vi "User_Login.vi"() -> ()   [LabVIEW 2020]
uses:
  <vilib>/Utility/cursorutil.llb/Set Cursor (Icon Pict).vi
panel:
  in  "Register":bool
  in  "Login":bool
  in  "User_Password":string caption="密    码"
  in  "User_Name":string caption="用户名"
  # "登录系统"
  # "@DTWAVES"
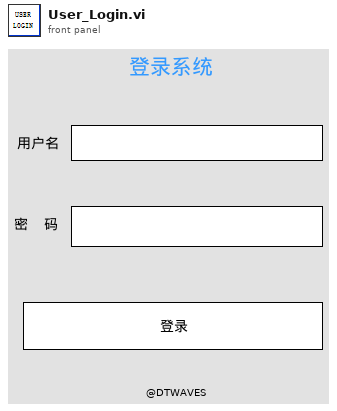
[diagram p1: front panel]
types:
  T1 = enum32{"Invalid", "Standard", "Closed", "Hidden", "Minimized", "Maximized"}
  T2 = enum32{"invalid app kind", "Development System", "Run Time System", "Student Edition", "Embedded LabVIEW", "Evaluation", "Custom"}
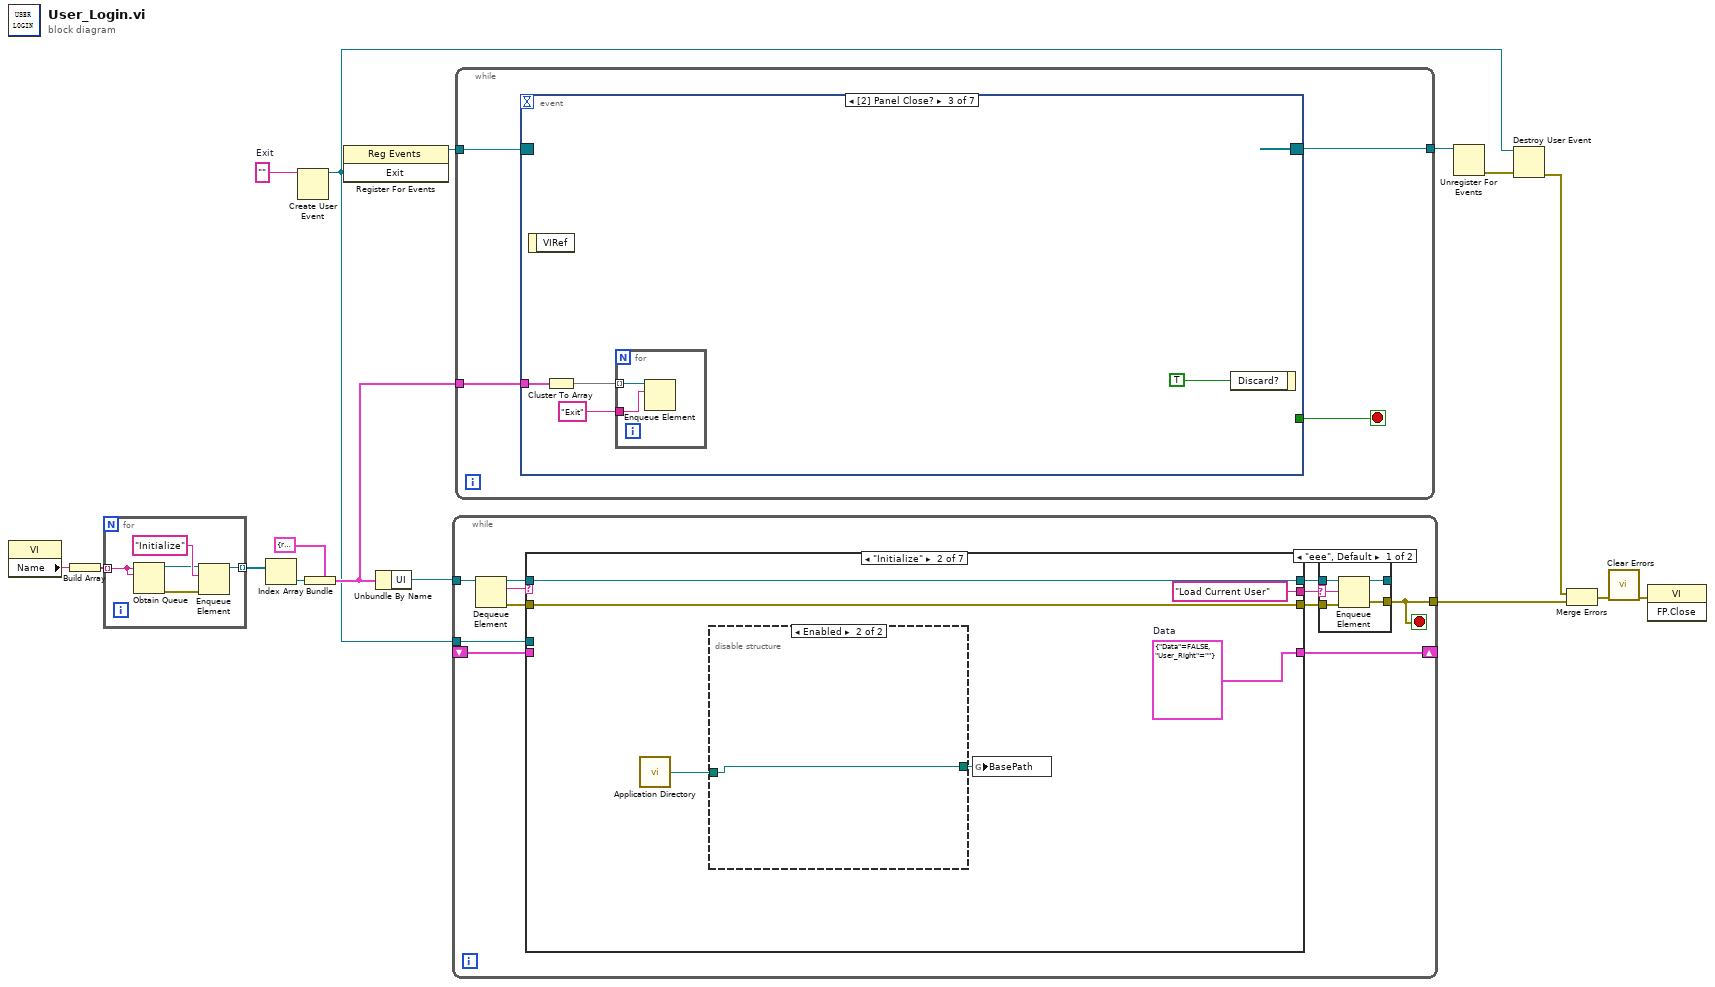
[diagram p0: block diagram]
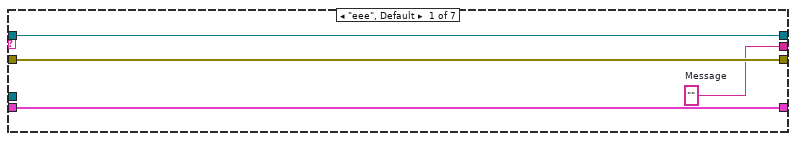
[diagram p3: hidden frame]
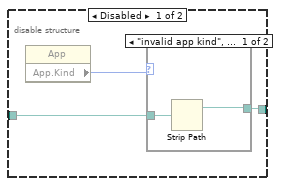
[diagram p4: hidden frame]
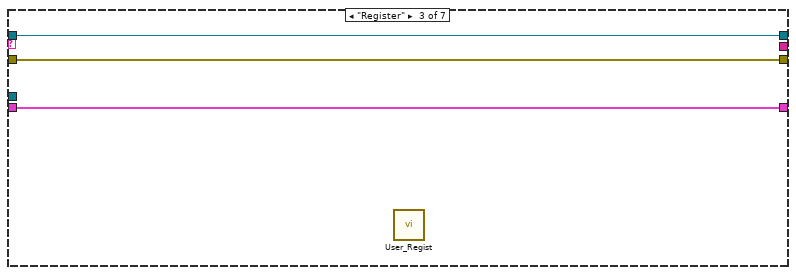
[diagram p6: hidden frame]
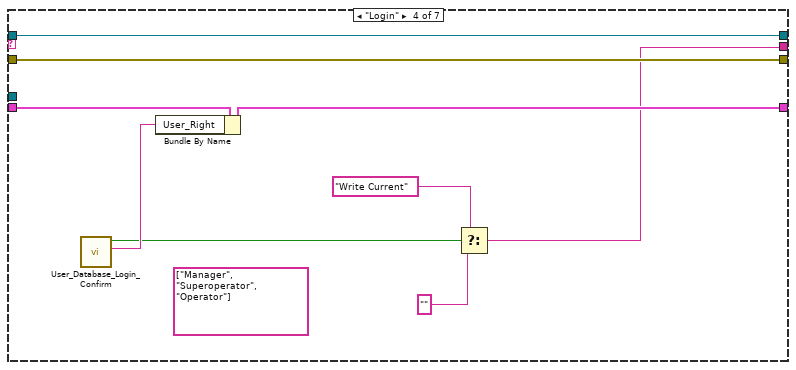
[diagram p7: hidden frame]
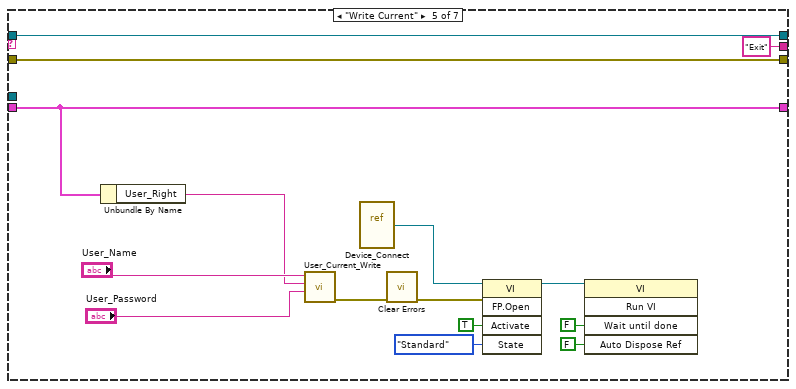
[diagram p8: hidden frame]
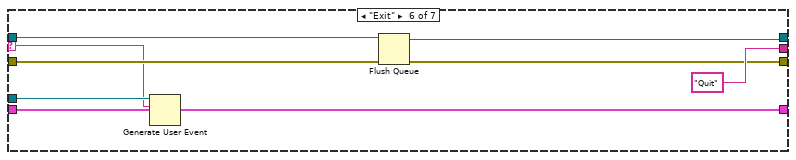
[diagram p9: hidden frame]
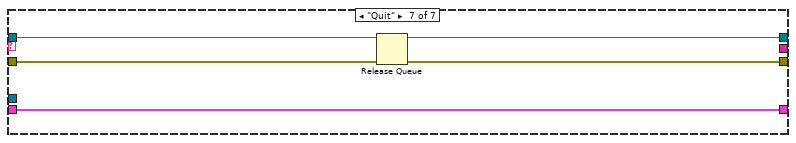
[diagram p10: hidden frame]
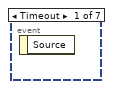
[diagram p11: hidden frame]
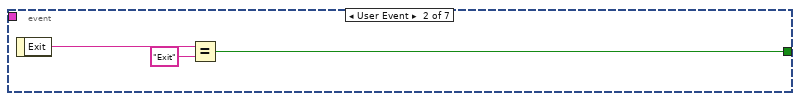
[diagram p12: hidden frame]
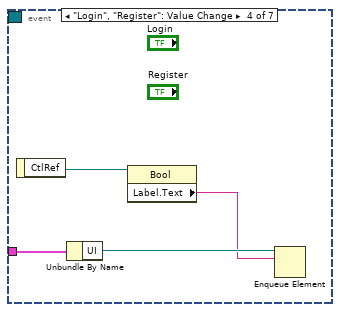
[diagram p13: hidden frame]
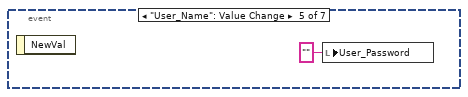
[diagram p14: hidden frame]
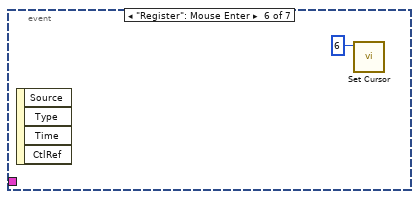
[diagram p15: hidden frame]
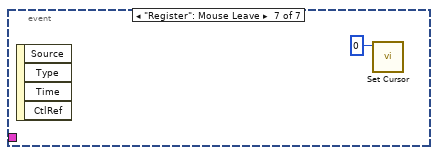
[diagram p16: hidden frame]
diagram:
  w2 = ""  # Exit
  n1 = property class="VI"() -> ("Name"=w12:string)  [unwired: 2 in, 2 out]
  n2 = Build Array(w12) -> (w13:string[])
  n3 = for {
    tunnel: w13 -> [w17] mode=indexing
    tunnel: [w18] -> w7 mode=indexing
    n4 = Obtain Queue(name (unnamed)=w17, element data type=w17) -> (queue out=w20:refnum<queue>, error out=w19:errorcluster)  [unwired: 3 in, 1 out]
    n5 = Enqueue Element(queue=w20, element="Initialize" ("元素"), error in (no error)=w19) -> (queue out=w18:refnum<queue>)  [unwired: 1 in, 2 out]
  }
  n6 = Index Array(array=w7) -> (element=w10:refnum<queue>)  [unwired: 1 in]
  n7 = Create User Event(user event datatype=w2) -> (user event=w6:refnum<user-event>)  [unwired: 1 in, 1 out]
  n8 = Bundle(cluster=cluster{"UI":refnum<queue>} {"UI"=refnum}, "UI"=w10) -> (w11:cluster{"UI":refnum<queue>})
  n9 = register-events(w6) -> (reference out=w3:refnum<event-registration>)  [unwired: 2 in, 1 out]
  n10 = Unbundle By Name(w11) -> ("UI"=w8:refnum<queue>)
  n11 = while {
    tunnel: w8 -> [w32]
    tunnel: [w22] -> w15
    shift-right: [w26] -> _
    shift-left: _ -> [w25]
    tunnel: w6 -> [w24]
    stop <- w22 stop-if-true
    n12 = Dequeue Element(queue=w32) -> (queue out=w31:refnum<queue>, element=w23:string, error out=w28:errorcluster)  [unwired: 2 in, 1 out]
    n13 = case shown="\"Initialize\"" w23 {
      selector: w23 -> [_ _ _ _ _ w84 _]
      tunnel: w31 -> [w43 w49 w59 w68 w83 w89 w95]
      tunnel: [w43 w49 w59 w68 w83 w88 w95] -> w30
      tunnel: [w42 w48 w58 w67 w82 w87 w92] -> w29
      tunnel: w28 -> [w42 w48 w58 w67 w82 w86 w94]
      tunnel: [w41 "Load Current User" ("Message") _ w60 "Exit" ("Message") "Quit" ("Message") _] -> w27
      tunnel: [w40 w47 w57 w65 w80 w91 w93] -> w26
      tunnel: w25 -> [w40 _ w57 w66 w80 w91 w93]
      tunnel: w24 -> [_ _ _ _ _ w85 _]
      frame "eee", Default {
        w41 = ""  # Message
      }
      frame "Initialize" {
        w47 = cluster{"Data":bool, "User_Right":string} {"Data"=FALSE, "User_Right"=""}  # Data
        n14 = call <vilib>:"Application Directory.vi"() -> ("Application Directory"=w45:path)
        n15 = disable-structure shown="Enabled" {
          disable-tunnel: w45 -> [w51 w56]
          disable-tunnel: [w50 w56] -> w44
          frame Disabled {
            n16 = property class="App"() -> ("App.Kind"=w52:T2)  [unwired: 2 in, 2 out]
            n17 = case shown="\"invalid app kind\", Default" w52 {
              tunnel: [w53 w55] -> w50
              tunnel: w51 -> [w54 w55]
              frame "invalid app kind", Default {
                n18 = Strip Path(path=w54) -> (stripped path=w53:path)  [unwired: 1 out]
              }
              frame "Development System" {
              }
            }
          }
          frame Enabled {
          }
        }
        n19 = global write "Global.vi" "BasePath"(w44) -> ()
      }
      frame "Register" {
        n20 = call "User_Regist.vi"() -> ()  [unwired: 12 in]
      }
      frame "Login" {
        (unwired) string[] ["Manager", "Superoperator", "Operator"] ("字符串数组")
        n21 = call "User_Database_Login_Confirm.vi"() -> ("User_Right"=w64:string, "OK"=w63:bool)  [unwired: 9 in, 1 out]
        n22 = Bundle By Name(cluster=w66, "User_Right"=w64) -> (w65:cluster{"Data":bool, "User_Right":string})
        n23 = Select(t="Write Current", s=w63, f="") -> (s? t:f=w60:string)
      }
      frame "Write Current" {
        n24 = Unbundle By Name(w80) -> ("User_Right"=w76:string)
        n25 = call "User_Current_Write.vi"("Password"="User_Password", "User_Right"=w76, "Name"="User_Name") -> ("error out"=w79:errorcluster)  [unwired: 8 in]
        n26 = vi-ref "Device_Connect.vi"() -> (w74:refnum<vi>)
        n27 = call <vilib>:"Clear Errors.vi"("error in (no error)"=w79) -> ("error out"=w69:errorcluster)  [unwired: 5 in, 1 out]
        n28 = invoke class="VI" method="FP.Open"(reference=w74, error in=w69, "Activate"=TRUE ("激活？"), "State"=T1."Standard" ("状态")) -> (reference out=w75:refnum<vi>)  [unwired: 1 in, 4 out]
        n29 = invoke class="VI" method="Run VI"(reference=w75, "Wait until done"=FALSE ("结束前等待"), "Auto Dispose Ref"=FALSE ("自动销毁引用")) -> ()  [unwired: 2 in, 5 out]
      }
      frame "Exit" {
        n30 = Generate User Event(user event=w85, event data cluster=w84) -> ()  [unwired: 2 in, 2 out]
        n31 = Flush Queue(queue=w89, error in (no error)=w86) -> (queue out=w88:refnum<queue>, error out=w87:errorcluster)  [unwired: 1 out]
      }
      frame "Quit" {
        n32 = Release Queue(queue=w95, error in (no error)=w94) -> (error out=w92:errorcluster)  [unwired: 1 in, 2 out]
      }
    }
    n33 = case shown="\"eee\", Default" w27 {
      selector: w27 -> [w33 _]
      tunnel: w30 -> [w37 w39]
      tunnel: w29 -> [w36 w38]
      tunnel: [w35 w38] -> w22
      tunnel: [w34 w39] -> _
      frame "eee", Default {
        n34 = Enqueue Element(queue=w37, element=w33, error in (no error)=w36) -> (queue out=w34:refnum<queue>, error out=w35:errorcluster)  [unwired: 1 in, 1 out]
      }
      frame "" {
      }
    }
  }
  n35 = while {
    tunnel: w3 -> [w98]
    tunnel: [w97] -> w5
    tunnel: w11 -> [w96]
    stop <- w99 stop-if-true
    n36 = event shown="[2] Panel Close?" {
      selector: w98 -> [_ _ _ _ _ _ _]
      dyn-events: [_ _ _ _ _ _ _] -> w97
      timeout: _ -> [_ _ _ _ _ _ _]
      tunnel: [_ w101 _ _ _ _ _] -> w99
      tunnel: w96 -> [_ _ w105 w112 _ _ _]
      event Timeout {
        n37 = event-data() -> ()  [unwired: 1 in, 1 out]
      }
      event User Event {
        n38 = event-data() -> ("Exit"=w102:string)  [unwired: 1 in]
        n39 = Equal?(x=w102, y="Exit") -> (x = y?=w101:bool)
      }
      event Panel Close? {
        n40 = event-data() -> ()  [unwired: 1 in, 1 out]
        n41 = Cluster To Array(cluster=w105) -> (array=w104:refnum<queue>[])
        n42 = for {
          tunnel: w104 -> [w108] mode=indexing
          tunnel: "Exit" ("元素") -> [w107]
          n43 = Enqueue Element(queue=w108, element=w107) -> ()  [unwired: 2 in, 3 out]
        }
        n44 = event-data("Discard?"=TRUE ("放弃？")) -> ()  [unwired: 1 in, 1 out]
      }
      event "Login", "Register": Value Change {
        n45 = event-data() -> ("CtlRef"=w110:refnum<vi>)  [unwired: 1 in]
        n46 = Unbundle By Name(w112) -> ("UI"=w111:refnum<queue>)
        n47 = property class="Bool"(reference=w110) -> ("Label.Text"=w109:string)  [unwired: 1 in, 2 out]
        n48 = Enqueue Element(queue=w111, element=w109) -> ()  [unwired: 2 in, 3 out]
      }
      event "User_Name": Value Change {
        n49 = event-data() -> ()  [unwired: 1 in, 1 out]
        n50 = local write "User_Password"("" ("User_Password")) -> ()
      }
      event "Register": Mouse Enter {
        n51 = event-data() -> ()  [unwired: 1 in, 4 out]
        n52 = call-poly <vilib>:"Set Cursor.vi"("icon"=u16 6) -> ()  [unwired: 9 in, 2 out]
      }
      event "Register": Mouse Leave {
        n53 = event-data() -> ()  [unwired: 1 in, 4 out]
        n54 = call-poly <vilib>:"Set Cursor.vi"("icon"=u16 0) -> ()  [unwired: 9 in, 2 out]
      }
    }
  }
  n55 = Unregister For Events(event registration refnum=w5) -> (error out=w4:errorcluster)  [unwired: 1 in]
  n56 = Destroy User Event(user event=w6, error in=w4) -> (error out=w14:errorcluster)
  n57 = Merge Errors(w14, w15) -> (w16:errorcluster)
  n58 = call <vilib>:"Clear Errors.vi"("error in (no error)"=w16) -> ("error out"=w1:errorcluster)  [unwired: 5 in, 1 out]
  n59 = invoke class="VI" method="FP.Close"(error in=w1) -> ()  [unwired: 2 in, 3 out]
